vi "Display Console View.vi"(8 "error in (no error)":errorcluster, 11 "View Model":T2) -> (0 "error out":errorcluster)   [LabVIEW 2017]
doc: "Display console for debugging elevator operation"
uses:
  View Model/Controls/View Model.ctl
  Error Handler/Controls/Error Model.ctl
  Error Handler/Controls/Error EventData.ctl
  Error Handler/Controls/Error Type.ctl
  Elevator Controller/Controls/Elevator Model.ctl
  Elevator Controller/Controls/Elevator Overhead.ctl
  Elevator Controller/Controls/Elevator States.ctl
  Elevator Controller/Controls/Elevator Location.ctl
  Elevator Controller/Controls/Elevator Command Event.ctl
  Elevator Controller/Controls/Elevator Commands.ctl
  Configuration/Controls/Configuration Model.ctl
  Configuration/Controls/Configuration Data.ctl
  View Model/Controls/Shared Model.ctl
panel:
  out "Emergency":bool
  out "Door Open":bool
  out "Down":bool
  out "Up":bool
  out "Elevator Location":T1
  out "Timing":dbl
  # "Elevator Direction"
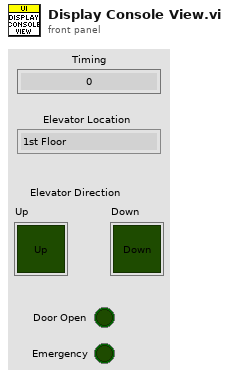
[diagram p1: front panel]
types:
  T1 = typedef "Elevator Location.ctl" = enum16{"1st Floor", "2nd Floor", "3rd Floor", "4th Floor"}
  T2 = typedef "View Model.ctl" = cluster{"Error Model":T3, "Elevator Model":T4, "Configuration Model":T5, "Shared Model":T6}
  T3 = typedef "Error Model.ctl" = cluster{"Error Event":refnum<user-event>}
  T4 = typedef "Elevator Model.ctl" = cluster{"Elevator Overhead":refnum<data-value>, "Floor Change":refnum<user-event>, "Elevator CMD":refnum<user-event>, "Motion Change":refnum<user-event>, "Direction Change":refnum<user-event>, "Door Position Change":refnum<user-event>, "Emergency Change":refnum<user-event>}
  T5 = typedef "Configuration Model.ctl" = cluster{"Config Change":refnum<user-event>, "Config DVR":refnum<data-value>}
  T6 = typedef "Shared Model.ctl" = cluster{"Stop DVR":refnum<data-value>, "Stop Event":refnum<user-event>}
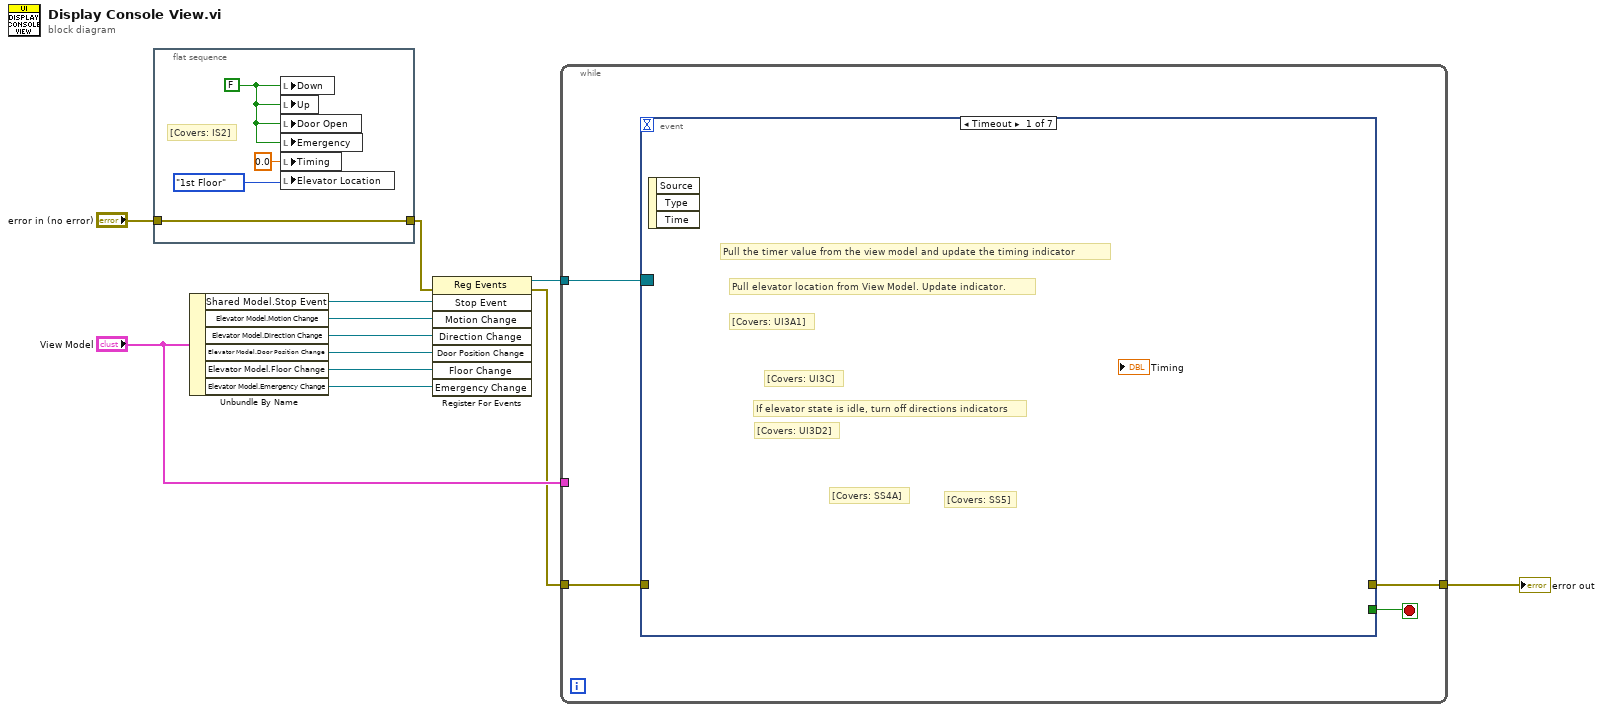
[diagram p0: block diagram]
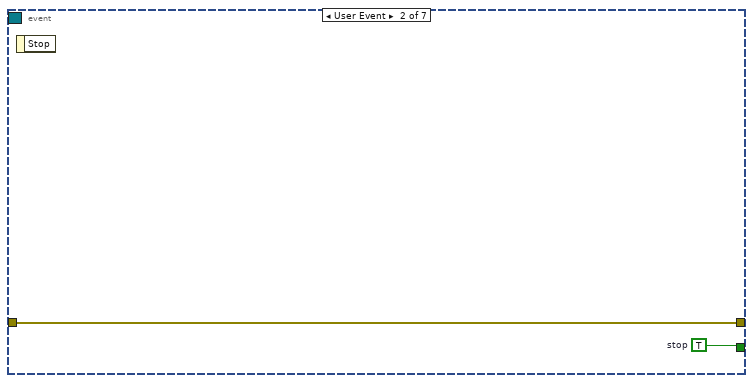
[diagram p2: hidden frame]
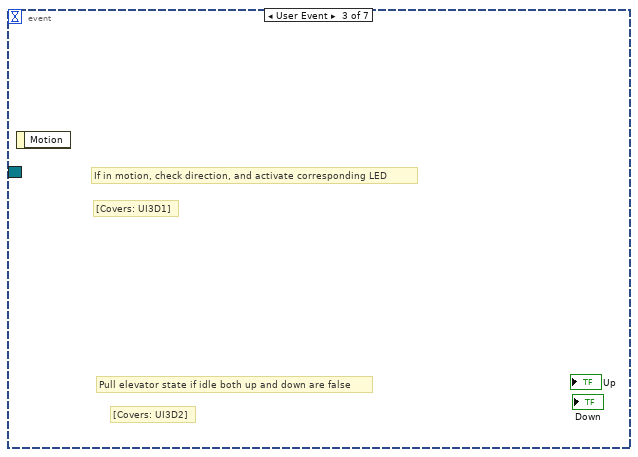
[diagram p3: hidden frame]
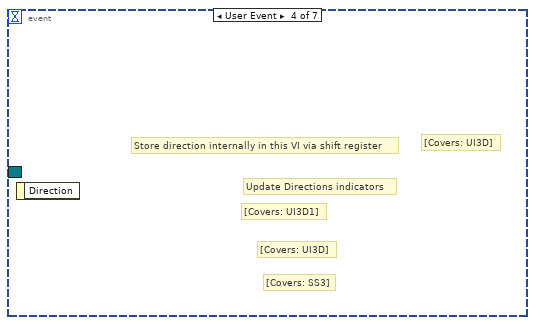
[diagram p4: hidden frame]
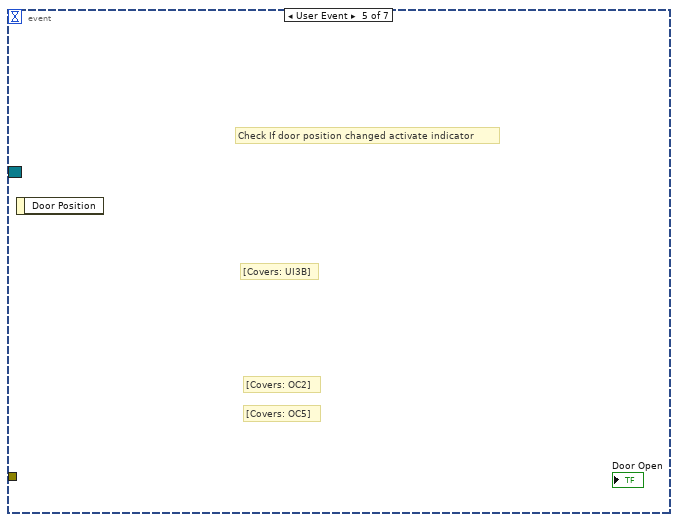
[diagram p5: hidden frame]
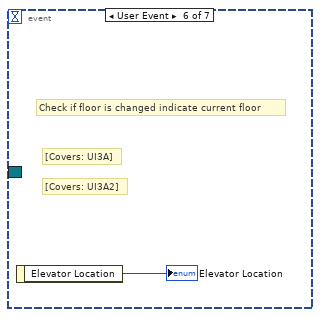
[diagram p6: hidden frame]
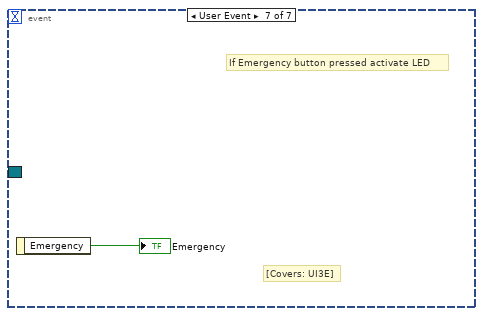
[diagram p7: hidden frame]
diagram:
  n1 = flat-sequence {
    tunnel: "error in (no error)" -> [w13]
    tunnel: [w13] -> w2
    frame #0 {
      w16 = FALSE ("Down")
      # "[Covers: IS2]"
      n2 = local write "Down"(w16) -> ()
      n3 = local write "Up"(w16) -> ()
      n4 = local write "Door Open"(w16) -> ()
      n5 = local write "Emergency"(w16) -> ()
      n6 = local write "Timing"(0.0 ("Timing")) -> ()
      n7 = local write "Elevator Location"(Elevator_Location."1st Floor" ("Elevator Location")) -> ()
    }
  }
  n8 = Unbundle By Name("View Model") -> ("Shared Model.Stop Event"=w12:refnum<user-event>, "Elevator Model.Motion Change"=w11:refnum<user-event>, "Elevator Model.Direction Change"=w5:refnum<user-event>, "Elevator Model.Door Position Change"=w6:refnum<user-event>, "Elevator Model.Floor Change"=w7:refnum<user-event>, "Elevator Model.Emergency Change"=w8:refnum<user-event>)
  n9 = register-events(error in=w2, w12, w11, w5, w6, w7, w8) -> (reference out=w10:refnum<event-registration>, error out=w1:errorcluster)  [unwired: 1 in]
  n10 = while {
    tunnel: w10 -> [w20]
    tunnel: w1 -> [w19]
    tunnel: [w18] -> w9
    tunnel: "View Model" -> [_]
    stop <- w17 stop-if-true
    n11 = event shown="[0] Timeout" {
      selector: w20 -> [_ _ _ _ _ _ _]
      dyn-events: _ -> [_ _ _ _ _ _ _]
      timeout: _ -> [_ _ _ _ _ _ _]
      tunnel: w19 -> [_ w22 _ _ _ _ _]
      tunnel: [_ w22 _ _ _ _ _] -> w18
      tunnel: [_ w21 _ _ _ _ _] -> w17
      event Timeout {
        # "[Covers: SS5]"
        # "[Covers: SS4A]"
        # "[Covers: UI3D2]"
        # "If elevator state is idle, turn off directions indicators"
        # "[Covers: UI3A1]"
        # "Pull elevator location from View Model. Update indicator."
        # "[Covers: UI3C]"
        # "Pull the timer value from the view model and update the timing indicator"
        n12 = event-data() -> ()  [unwired: 1 in, 3 out]
      }
      event User Event {
        w21 = TRUE  # stop
        n13 = event-data() -> ()  [unwired: 1 in, 1 out]
      }
      event User Event {
        # "[Covers: UI3D2]"
        # "Pull elevator state if idle both up and down are false"
        # "[Covers: UI3D1]"
        # "If in motion, check direction, and activate corresponding LED"
        n14 = event-data() -> ()  [unwired: 1 in, 1 out]
      }
      event User Event {
        # "[Covers: SS3]"
        # "[Covers: UI3D]"
        # "[Covers: UI3D1]"
        # "Update Directions indicators"
        # "[Covers: UI3D]"
        # "Store direction internally in this VI via shift register"
        n15 = event-data() -> ()  [unwired: 1 in, 1 out]
      }
      event User Event {
        # "[Covers: OC5]"
        # "[Covers: OC2]"
        # "[Covers: UI3B]"
        # "Check If door position changed activate indicator"
        n16 = event-data() -> ()  [unwired: 1 in, 1 out]
      }
      event User Event {
        # "[Covers: UI3A2]"
        # "[Covers: UI3A]"
        # "Check if floor is changed indicate current floor"
        n17 = event-data() -> ("Elevator Location"=→"Elevator Location":T1)  [unwired: 1 in]
      }
      event User Event {
        # "[Covers: UI3E]"
        # "If Emergency button pressed activate LED"
        n18 = event-data() -> ("Emergency"=→"Emergency":bool)  [unwired: 1 in]
      }
    }
  }
  "error out" <- w9
